vi "Calculate Jacobian.vi"(8 "Error In":errorcluster, 10 "RProp Data":T1={"Empty Gradient"=[], "Gradient Register"=[], "Teach Coef Register"=[], "Current Gradient"=[], "# Vectors per Iteration"=2, "Teaching Set Ref"=refnum, "Validation Set Ref"=refnum, "Error Buffer"=[], "# Samples"=0, "Gradient Sign Running Value"=[]}, 11 "Neural Network In":refnum<class "Neural Network.lvclass">) -> (0 "Error Out":errorcluster, 1 "Total % Error / Output":dbl[](array[numeric]), 2 "RProp Data Out":T1={"Empty Gradient"=[], "Gradient Register"=[], "Teach Coef Register"=[], "Current Gradient"=[], "# Vectors per Iteration"=2, "Teaching Set Ref"=refnum, "Validation Set Ref"=refnum, "Error Buffer"=[], "# Samples"=0, "Gradient Sign Running Value"=[]}, 3 "Neural Network Out":refnum<class "Neural Network.lvclass">)   [LabVIEW 2015, in "Neural Network.lvclass"]
uses:
  Neural Network.lvclass
  Teaching File/Teaching File.lvlib
  Types/2D Array.ctl
  Types/RProp Algorithm.ctl
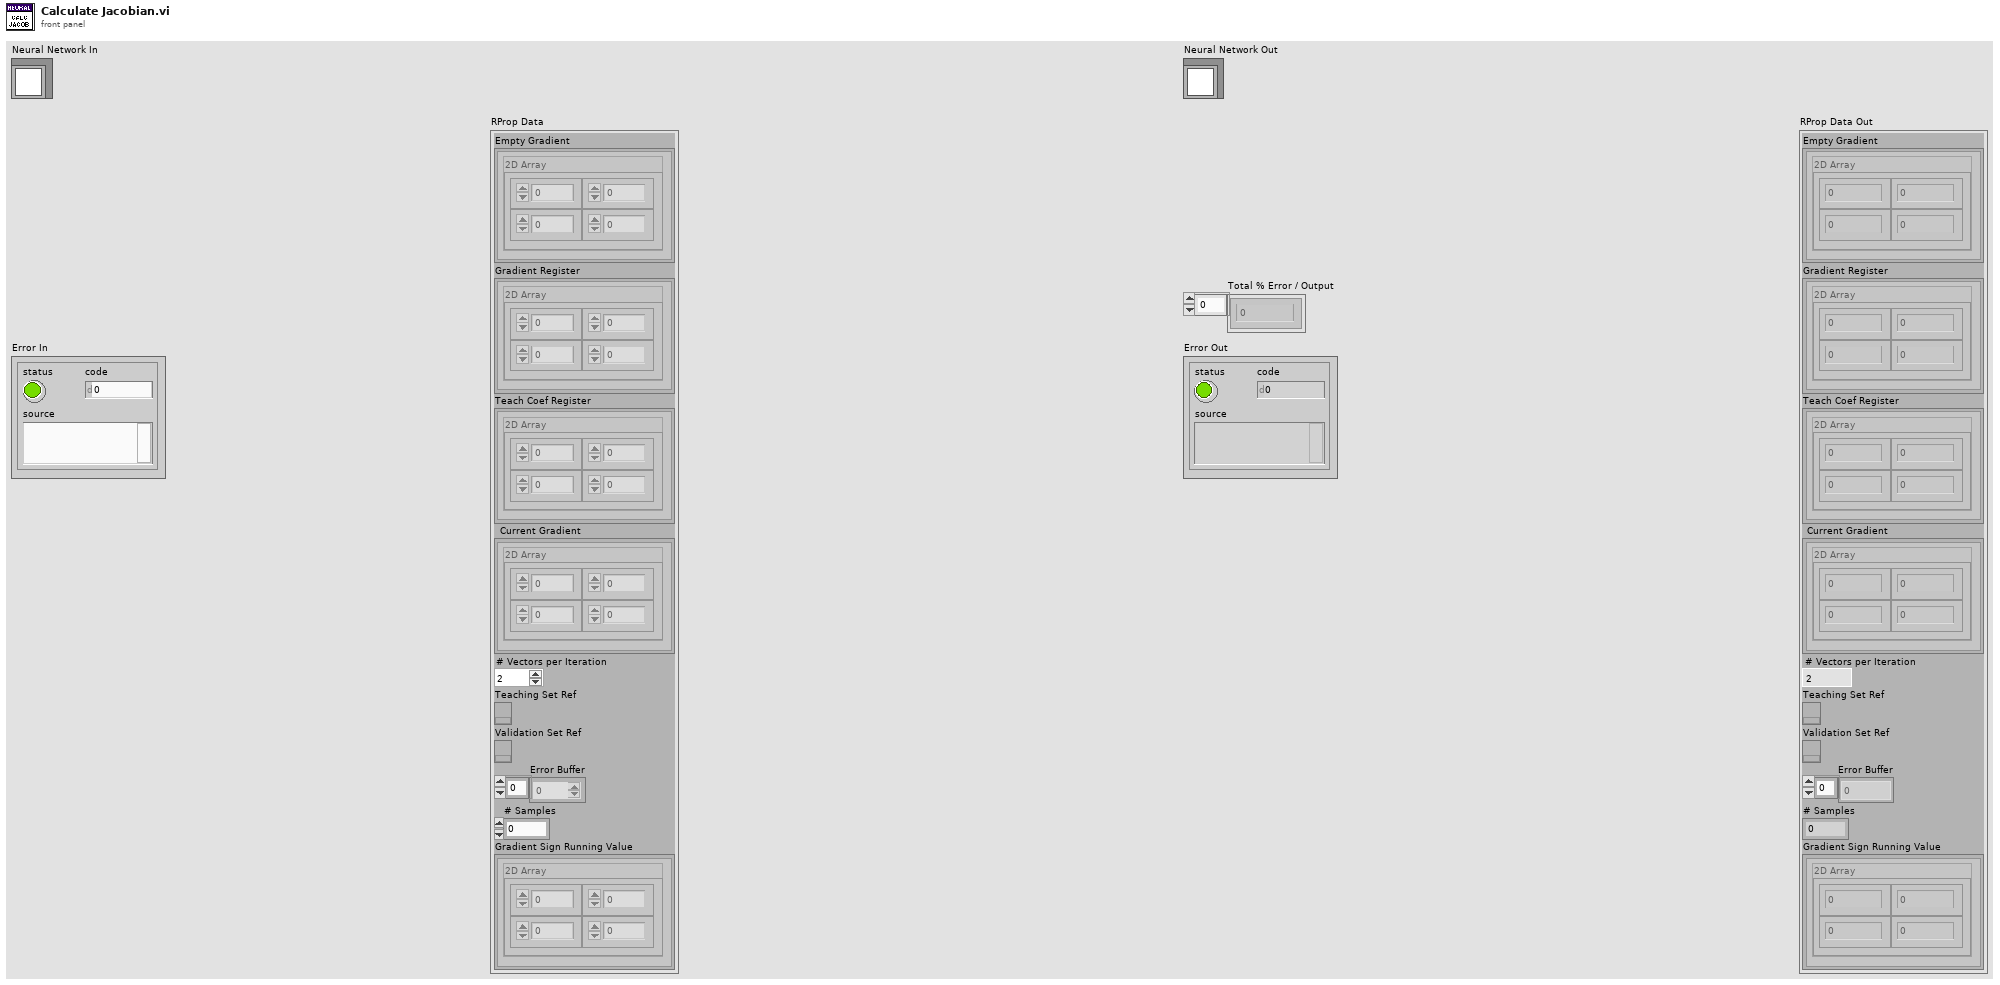
[diagram p1: front panel]
types:
  T1 = typedef "Neural Network.lvclass/RProp Algorithm.ctl" = cluster{"Empty Gradient":T2[], "Gradient Register":T2[], "Teach Coef Register":T2[], "Current Gradient":T2[], "# Vectors per Iteration":i64, "Teaching Set Ref":refnum<k34>, "Validation Set Ref":refnum<k34>, "Error Buffer":dbl[], "# Samples":i64, "Gradient Sign Running Value":T2[]}
  T2 = typedef "Neural Network.lvclass/2D Array.ctl" = cluster{"2D Array":sgl[][]}
  T3 = typedef "Neural Network.lvclass/Scaling Info.ctl" = cluster{"X Scaling Vector":dbl[], "Y Scaling Vector":dbl[]}
  T4 = typedef "Neural Network.lvclass/1D Array.ctl" = cluster{"1D Array":dbl[]}
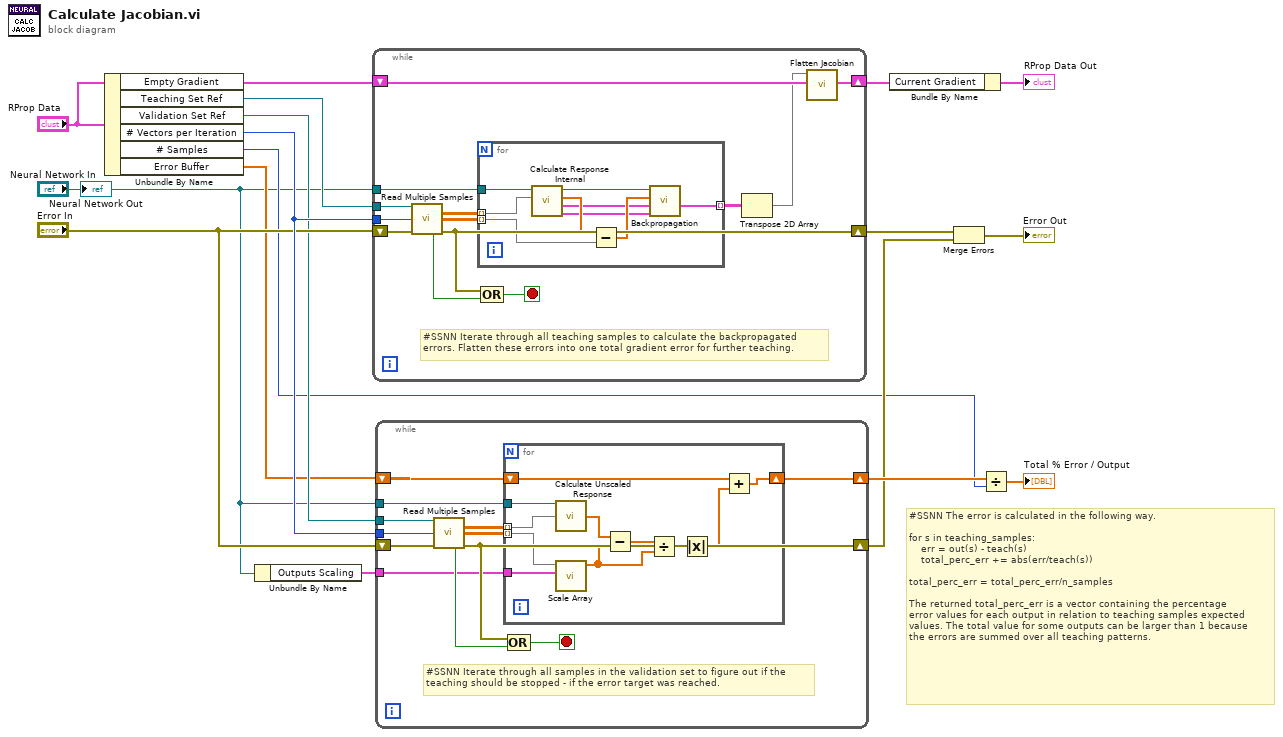
[diagram p0: block diagram]
diagram:
  # "#SSNN The error is calculated in the following way.\n\nfor s in teaching_samples:\n    err = out(s) - teach(s)\n    total_perc_err += abs(err/teach(s))\n\ntotal_perc_err = total_perc_err/n_samples\n\nThe returned total_perc_err is a vector containing the percentage\nerror values for each output in relation to teaching samples expected\nvalues. The total value for some outputs can be larger than 1 because\nthe errors are summed over all teaching patterns."
  n1 = Unbundle By Name("RProp Data") -> ("Empty Gradient"=w14:T2[], "Teaching Set Ref"=w11:refnum<k34>, "Validation Set Ref"=w5:refnum<k34>, "# Vectors per Iteration"=w10:i64, "# Samples"=w4:i64, "Error Buffer"=w3:dbl[])
  n2 = Unbundle By Name("Neural Network In") -> ("Outputs Scaling"=w1:T3)
  n3 = while {
    tunnel: "Neural Network In" -> [w30]
    shift-right: [w26] -> w13
    shift-left: w14 -> [w28]
    tunnel: w11 -> [w23]
    tunnel: w10 -> [w18]
    shift-right: [w20] -> w12
    shift-left: "Error In" -> [w22]
    stop <- w19 stop-if-true
    # "#SSNN Iterate through all teaching samples to calculate the backpropagated\nerrors. Flatten these errors into one total gradient error for further teaching."
    # "Iterate through all teaching samples in chunks \nand flatten the Jacobian into GRADIENT on chunk basis"
    n4 = call "Read Multiple Samples.vi"("TDMS In"=w23, "#samples (-1: all)"=w18, "Error In"=w22) -> ("Input Vectors"=w25:dbl[][], "Output Vectors"=w24:dbl[][], "EOF?"=w21:bool, "Error Out"=w20:errorcluster)  [unwired: 8 in, 1 out]
    n5 = for {
      tunnel: [w34] -> w29 mode=indexing
      tunnel: w30 -> [w38]
      tunnel: w25 -> [w32] mode=indexing
      tunnel: w24 -> [w31] mode=indexing
      # "Parallelized to use all cores"
      n6 = call "Calculate Response Internal.vi"("Inputs"=w32, "Neural Network In"=w38) -> ("All Inputs"=w35:T4[], "Derrivatives"=w36:T4[], "Outputs"=w39:dbl[], "Neural Network Out"=w33:refnum<class "Neural Network.lvclass">)  [unwired: 6 in]
      n7 = Subtract(x=w39, y=w31) -> (x-y=w37:dbl[])
      n8 = call "Backpropagation.vi"("All Inputs"=w35, "Derrivatives"=w36, "Error"=w37, "Neural Network In"=w33) -> ("Gradient Out"=w34:T2[])  [unwired: 7 in]
    }
    n9 = Compound Arithmetic op=OR(w20, w21) -> (w19:bool)
    n10 = Transpose 2D Array(2D array=w29) -> (transposed array=w27:T2[][])
    n11 = call "Flatten Jacobian.vi"("Gradient In"=w28, "Jacobian"=w27) -> ("Gradient Out"=w26:T2[])  [unwired: 9 in]
  }
  n12 = while {
    tunnel: "Neural Network In" -> [w51]
    tunnel: w10 -> [w47]
    shift-right: [w45] -> w7
    shift-left: "Error In" -> [w48]
    shift-right: [w42] -> w8
    shift-left: w3 -> [w43]
    tunnel: w5 -> [w41]
    tunnel: w1 -> [w40]
    stop <- w44 stop-if-true
    # "#SSNN Iterate through all samples in the validation set to figure out if the\nteaching should be stopped - if the error target was reached."
    # "Iterate through all teaching samples in chunks and flatten the Jacobian into GRADIENT on chunk basis"
    n13 = call "Read Multiple Samples.vi"("TDMS In"=w41, "#samples (-1: all)"=w47, "Error In"=w48) -> ("Input Vectors"=w50:dbl[][], "Output Vectors"=w49:dbl[][], "EOF?"=w46:bool, "Error Out"=w45:errorcluster)  [unwired: 8 in, 1 out]
    n14 = for {
      tunnel: w51 -> [w55]
      tunnel: w50 -> [w52] mode=indexing
      tunnel: w49 -> [w54] mode=indexing
      shift-right: [w60] -> w42
      shift-left: w43 -> [w61]
      tunnel: w40 -> [w56]
      # "Parallelized to use all cores"
      n15 = call "Calculate Unscaled Response.vi"("Neural Network In"=w55, "Inputs"=w52) -> ("Unscaled Outputs"=w53:dbl[])  [unwired: 11 in, 2 out]
      n16 = call "Scale Array.vi"("Scaling Info"=w56, "Array to Scale"=w54) -> ("Scaled Array"=w57:dbl[])  [unwired: 9 in]
      n17 = Subtract(x=w53, y=w57) -> (x-y=w62:dbl[])
      n18 = Divide(x=w62, y=w57) -> (x/y=w59:dbl[])
      n19 = Absolute Value(x=w59) -> (abs(x)=w58:dbl[])
      n20 = Add(x=w61, y=w58) -> (x+y=w60:dbl[])
    }
    n21 = Compound Arithmetic op=OR(w45, w46) -> (w44:bool)
  }
  n22 = Bundle By Name(cluster="RProp Data", "Current Gradient"=w13) -> (→"RProp Data Out":T1)
  n23 = Merge Errors(w12, w7) -> (→"Error Out":errorcluster)
  n24 = Divide(x=w8, y=w4) -> (x/y=→"Total % Error / Output":dbl[])
  "Neural Network Out" <- "Neural Network In"
